vi "LCVR Output.vi"(9 "Ch index":i16, 10 "V index":i16, 11 "Voltages":dbl[][](array[numeric]) format="%0.3f") -> ()   [LabVIEW 2012]
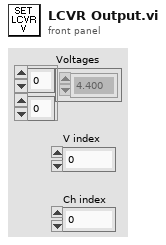
[diagram p1: front panel]
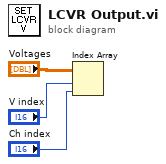
[diagram p0: block diagram]
diagram:
  n1 = Index Array(array="Voltages", index (row)="V index", index (col)="Ch index") -> ()  [unwired: 1 out]
